vi "Generate HHP.vi"(8 "error in (no error)":errorcluster, 11 "CHM Generator in":refnum<class "CHM Generator.lvclass">) -> (0 "error out":errorcluster, 3 "CHM Generator out":refnum<class "CHM Generator.lvclass">)   [LabVIEW 2020, in "CHM Generator.lvclass"]
uses:
  CHM Generator.lvclass
  CHM Generator.lvclass/CHM Generator.ctl
  Keyed Value Tree/Keyed Value Tree.lvclass
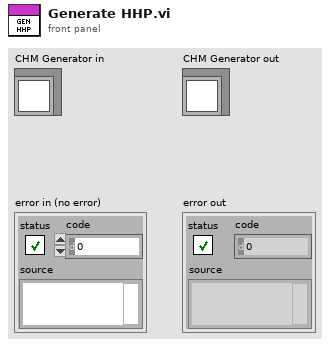
[diagram p1: front panel]
types:
  T1 = enum16{"open", "replace", "create", "open or create", "replace or create", "replace or create with confirmation"}
  T2 = typedef "Keyed Value Tree.lvclass/Keyed Value Pair.ctl" = cluster{"Key":string, "Value":string}
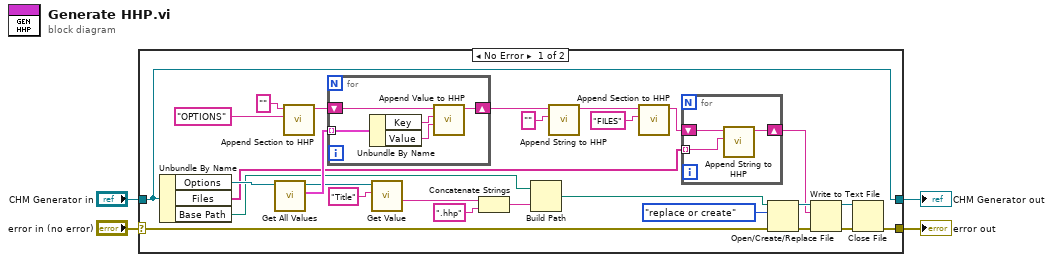
[diagram p0: block diagram]
diagram:
  n1 = case shown="No Error" "error in (no error)" {
    selector: "error in (no error)" -> [w16 w41]
    tunnel: [w15 w41] -> w3
    tunnel: [w29 w40] -> w1
    tunnel: "CHM Generator in" -> [w29 w40]
    frame No Error {
      n2 = Unbundle By Name(w29) -> ("Options"=w28:refnum<class "Keyed Value Tree.lvclass">, "Files"=w24:string[], "Base Path"=w10:path)
      n3 = call-dynamic "Get All Values.vi"("Keyed Value Tree in"=w28) -> ("Keyed Value Pairs"=w27:T2[], "Keyed Value Tree out"=w11:refnum<class "Keyed Value Tree.lvclass">)  [unwired: 8 in, 1 out]
      n4 = call "Append Section to HHP.vi"("Value"="OPTIONS", "HHP String In"="") -> ("HHP String Out"=w26:string)  [unwired: 9 in]
      n5 = for {
        tunnel: w27 -> [w39] mode=indexing
        shift-right: [w37] -> w14
        shift-left: w26 -> [w38]
        n6 = Unbundle By Name(w39) -> ("Key"=w36:string, "Value"=w35:string)
        n7 = call "Append Value to HHP.vi"("Value"=w35, "Key"=w36, "HHP String In"=w38) -> ("HHP String Out"=w37:string)  [unwired: 8 in]
      }
      n8 = call-dynamic "Get Value.vi"("name"="Title", "Keyed Value Tree in"=w11) -> ("value"=w5:string)  [unwired: 6 in, 3 out]
      n9 = Concatenate Strings(w5, ".hhp" ("element")) -> (w6:string)
      n10 = Build Path(base path=w10, name or relative path=w6) -> (appended path=w9:path)
      n11 = call "Append String to HHP.vi"("Value"="", "HHP String In"=w14) -> ("HHP String Out"=w13:string)  [unwired: 9 in]
      n12 = call "Append Section to HHP.vi"("Value"="FILES", "HHP String In"=w13) -> ("HHP String Out"=w23:string)  [unwired: 9 in]
      n13 = for {
        tunnel: w24 -> [w34] mode=indexing
        shift-right: [w32] -> w19
        shift-left: w23 -> [w33]
        n14 = call "Append String to HHP.vi"("Value"=w34, "HHP String In"=w33) -> ("HHP String Out"=w32:string)  [unwired: 9 in]
      }
      n15 = Open/Create/Replace File(file path (use dialog)=w9, error in=w16, operation (0:open)=T1."replace or create") -> (refnum out=w20:refnum<file>, error out=w21:errorcluster)  [unwired: 3 in, 1 out]
      n16 = Write to Text File(file (use dialog)=w20, text=w19, error in=w21) -> (refnum out=w17:refnum<file>, error out=w18:errorcluster)  [unwired: 1 in, 1 out]
      n17 = Close File(refnum=w17, error in=w18) -> (error out=w15:errorcluster)  [unwired: 1 out]
    }
    frame Error {
    }
  }
  "error out" <- w3
  "CHM Generator out" <- w1
